vi "メイン_装飾移動サブ.vi"(8 "Y軸座標入力":dbl, 11 "VI入力":refnum<vi>) -> ()   [LabVIEW 2021]
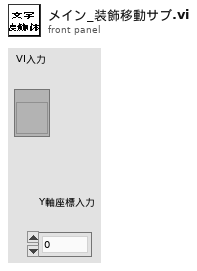
[diagram p1: front panel]
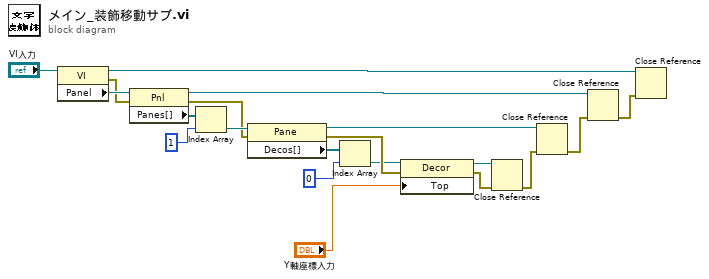
[diagram p0: block diagram]
diagram:
  n1 = property class="VI"(reference="VI入力") -> (reference out=w6:refnum<vi>, error out=w12:errorcluster, "Panel"=w17:refnum<vi>)  [unwired: 1 in]
  n2 = property class="Pnl"(reference=w17, error in=w12) -> (reference out=w7:refnum<vi>, error out=w11:errorcluster, "Panes[]"=w18:refnum<vi>[])
  n3 = Index Array(array=w18, index=1) -> (element=w20:refnum<vi>)
  n4 = property class="Pane"(reference=w20, error in=w11) -> (reference out=w8:refnum<vi>, error out=w16:errorcluster, "Decos[]"=w13:refnum<vi>[])
  n5 = Index Array(array=w13, index=0) -> (element=w15:refnum<vi>)
  n6 = property class="Decor"(reference=w15, error in=w16, "Top"="Y軸座標入力") -> (reference out=w9:refnum<vi>, error out=w5:errorcluster)
  n7 = Close Reference(reference=w9, error in (no error)=w5) -> (error out=w4:errorcluster)
  n8 = Close Reference(reference=w8, error in (no error)=w4) -> (error out=w3:errorcluster)
  n9 = Close Reference(reference=w7, error in (no error)=w3) -> (error out=w2:errorcluster)
  n10 = Close Reference(reference=w6, error in (no error)=w2) -> ()  [unwired: 1 out]
